vi "Diagnose.vi"(8 "error in (no error)":errorcluster, 11 "Slave Address":i32) -> (0 "error out":errorcluster, 2 "Command":string)   [LabVIEW 2014, in "Modbus.lvlib"]
uses:
  Modbus.lvlib
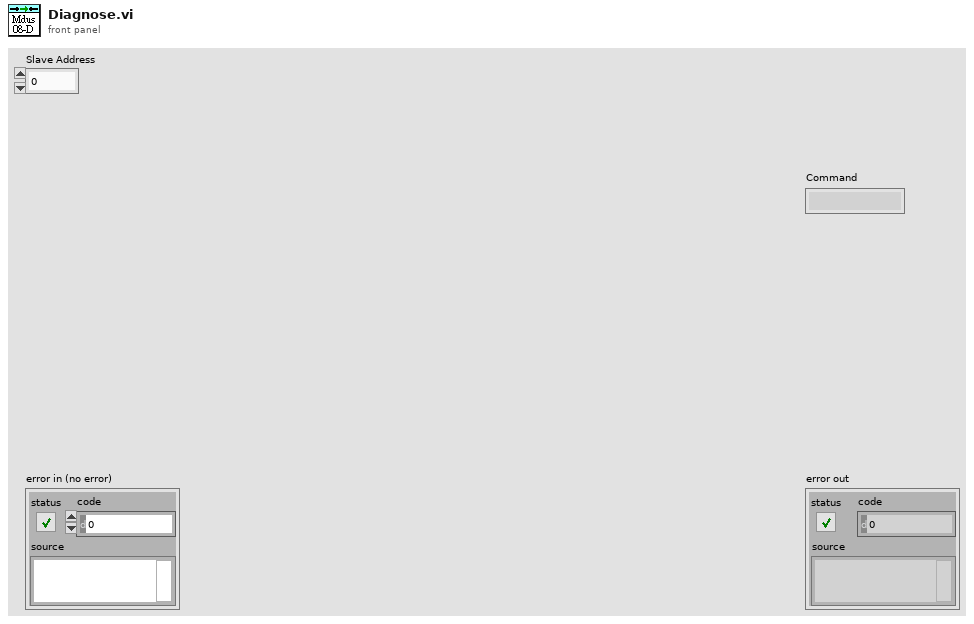
[diagram p1: front panel]
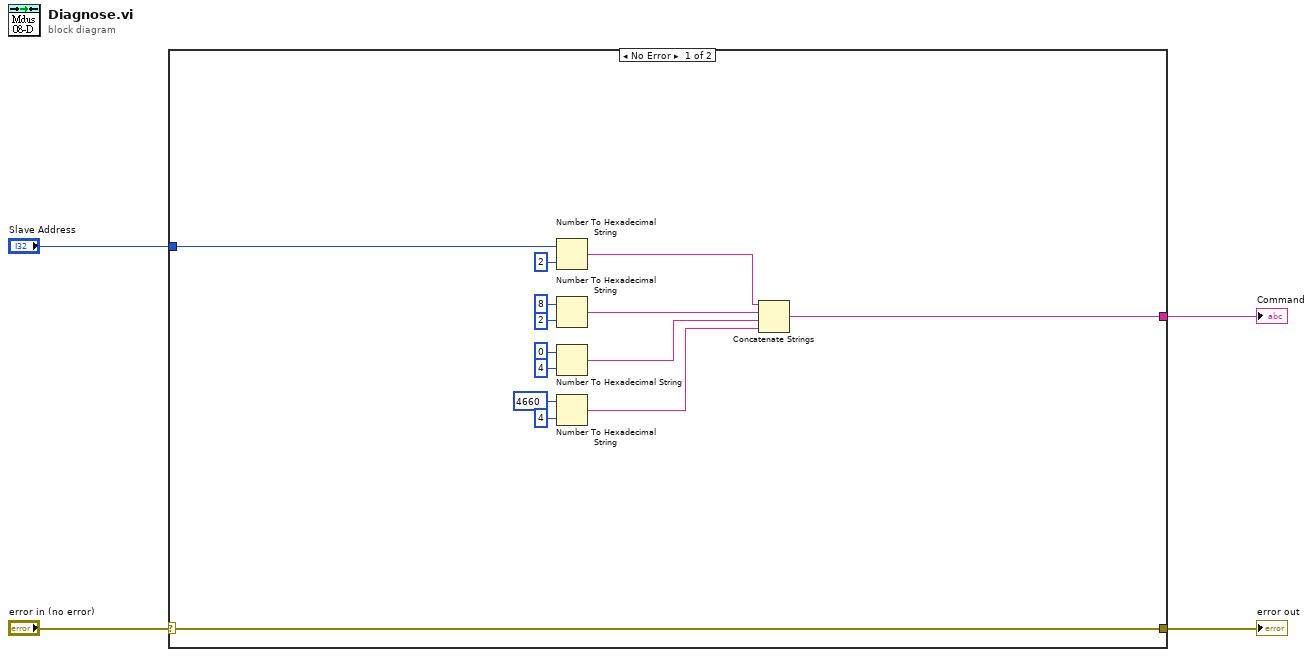
[diagram p0: block diagram]
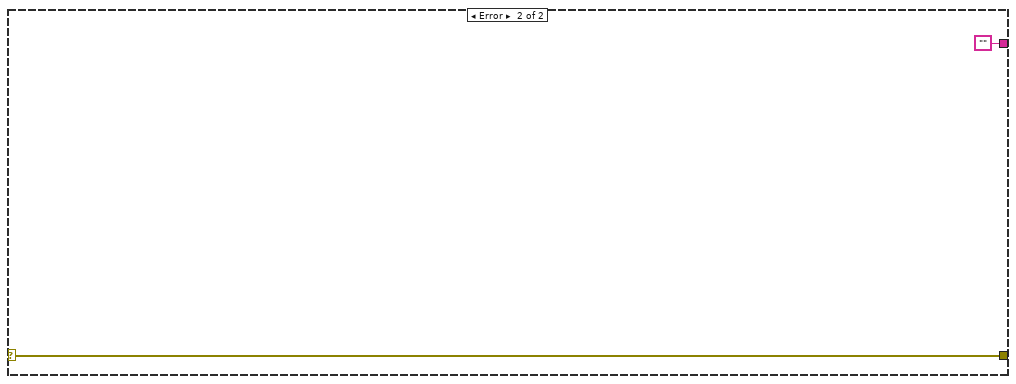
[diagram p2: hidden frame]
diagram:
  n1 = case shown="No Error" "error in (no error)" {
    selector: "error in (no error)" -> [w18 w20]
    tunnel: [w18 w20] -> w3
    tunnel: "Slave Address" -> [w6 _]
    tunnel: [w5 ""] -> w1
    frame No Error {
      n2 = Number To Hexadecimal String(1:i16 2 ("width (-)"), 2:w6) -> (0:w13:string)
      n3 = Number To Hexadecimal String(1:i16 2 ("width (-)"), 2:8 ("number")) -> (0:w12:string)
      n4 = Number To Hexadecimal String(1:i16 4 ("width (-)"), 2:0 ("number")) -> (0:w11:string)
      n5 = Number To Hexadecimal String(1:i16 4 ("width (-)"), 2:4660 ("number")) -> (0:w9:string)
      n6 = Concatenate Strings(w13, w12, w11, w9) -> (w5:string)
    }
    frame Error {
    }
  }
  "error out" <- w3
  "Command" <- w1
